vi "DAQ DI.vi"(8 "error in":errorcluster, 11 "Alias":string) -> (0 "error out":errorcluster, 3 "DI out":bool)   [LabVIEW 2021]
uses:
  Load INI/Controls/DAQ_Data.ctl
  <vilib>/DAQmx/read.llb/DAQmx Read (Digital Bool 1Line 1Point).vi
  <vilib>/DAQmx/create/channels.llb/DAQmx Create Channel (DI-Digital Input).vi
  <vilib>/DAQmx/miscellaneous.llb/DAQmx Fill In Error Info.vi
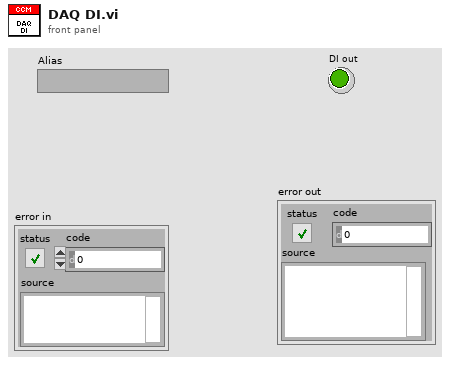
[diagram p1: front panel]
types:
  T1 = typedef "DAQ_Data.ctl" = cluster{"Alias":string, "DAQ Ch":string}
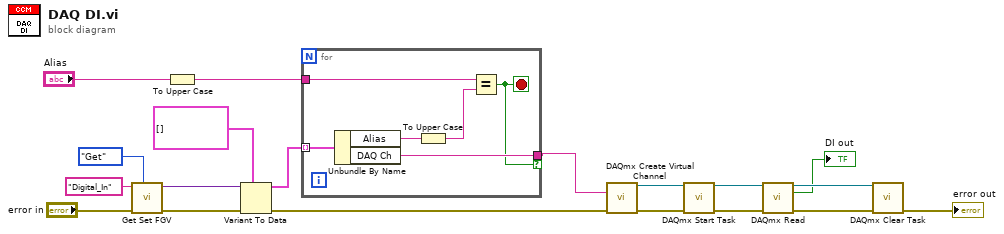
[diagram p0: block diagram]
diagram:
  n1 = call "Get Set FGV.vi"("Method (Get)"=enum16{"Get", "Set"}."Get", "error in"="error in", "Name"="Digital_In") -> ("error out"=w11:errorcluster, "Data out"=w10:variant)  [unwired: 7 in]
  n2 = To Upper Case(1:"Alias") -> (0:w2:string)
  n3 = Variant To Data(error in=w11, type=T1[] [], Variant=w10) -> (data=w5:T1[], error out=w7:errorcluster)
  n4 = for {
    tunnel: w5 -> [w25] mode=indexing
    tunnel: [w24] -> w3 if=w21
    tunnel: w2 -> [w23]
    stop <- w21 stop-if-true
    n5 = Unbundle By Name(w25) -> ("Alias"=w22:string, "DAQ Ch"=w24:string)
    n6 = To Upper Case(1:w22) -> (0:w20:string)
    n7 = Equal?(x=w23, y=w20) -> (x = y?=w21:bool)
  }
  n8 = call-poly <vilib>:"DAQmx Create Virtual Channel.vi"("lines"=w3, "error in"=w7) -> ("task out"=w15:refnum<k21>, "error out"=w16:errorcluster)  [unwired: 12 in]
  n9 = call <vilib>:"DAQmx Start Task.vi"("task/channels in"=w15, "error in"=w16) -> ("task out"=w18:refnum<k21>, "error out"=w17:errorcluster)  [unwired: 12 in]
  n10 = call-poly <vilib>:"DAQmx Read.vi"("task/channels in"=w18, "error in"=w17) -> ("task out"=w14:refnum<k21>, "data"=→"DI out":bool, "error out"=w13:errorcluster)  [unwired: 11 in]
  n11 = call <vilib>:"DAQmx Clear Task.vi"("task in"=w14, "error in"=w13) -> ("error out"=→"error out":errorcluster)  [unwired: 13 in]
